vi "Image Browser.vi"() -> ()   [LabVIEW 2014]
doc: "This example shows how to set up an image browser. An image browser is a concise representation of the images in your database represented as thumbnails on a page. You can use the Browser VIs in NI Vision to configure a browser, configure the selection of one or many images, add new images and remove images to and from a browser, replace an image, and get or set the selection status of an image."
uses:
  <vilib>/vision/NI_Vision_Development_Module.lvlib
panel:
  out "Image":T1(plugin-control)
  in  "Stop":bool
  # "Overview: Demonstrates how to use the IMAQ Browser functions to display multiple thumbnail images in a single display. and allow the user to select images from the browser.\nRequirements: Vision Development Software.\nInstructions:\n1. Run the VI.\n2. Click on the images to select or unselect them."
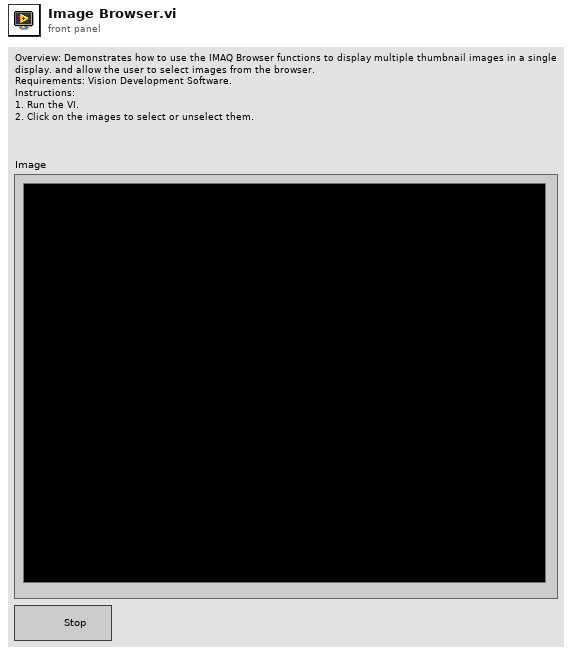
[diagram p1: front panel]
types:
  T1 = typedef "IMAQ Image.ctl" = refnum<image>
  T2 = cluster{"Browser Size":cluster{"X":i32, "Y":i32}, "Images per Line":i32, "Background Color":u32, "Frame Size":i32, "Frame Style":u16}
  T3 = typedef "Image Type" = u32
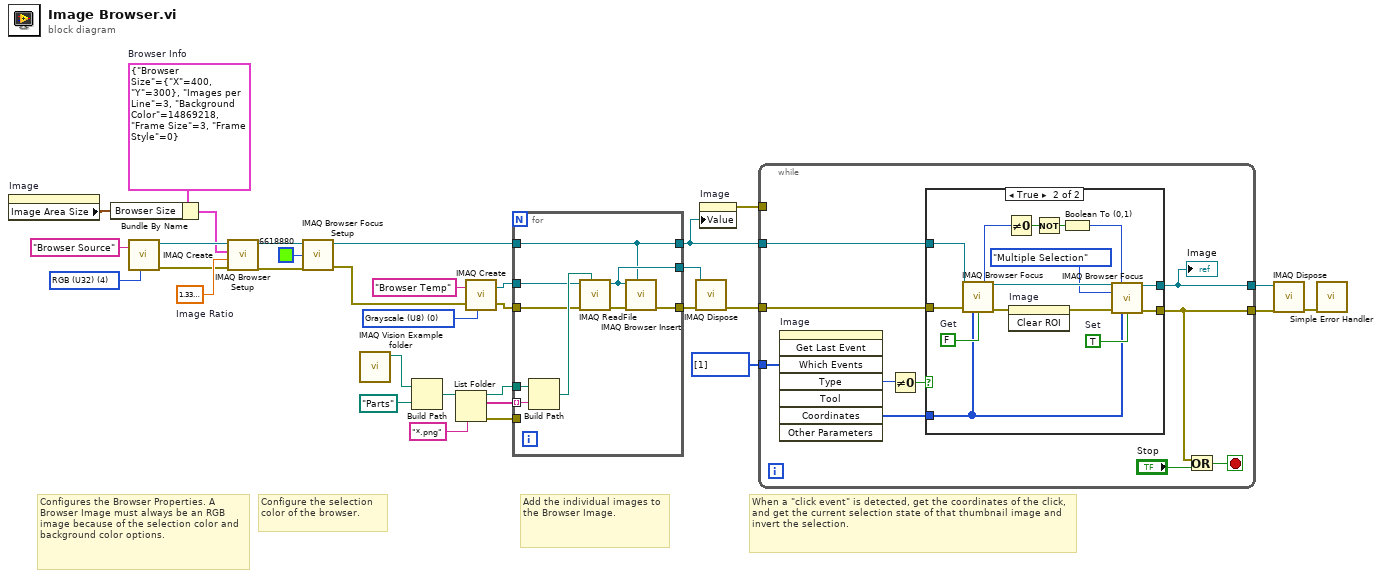
[diagram p0: block diagram]
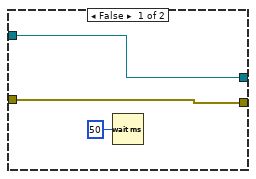
[diagram p2: hidden frame]
diagram:
  w17 = i32[] [1] items=["No Event"=0, "Click Event"=1, "Draw Event"=2, "Size Event"=4, "Scroll Event"=5, "Double Click Event"=8] ("Which Events")
  w33 = sgl 1.33  # Image Ratio
  w5 = T2 {"Browser Size"={"X"=400, "Y"=300}, "Images per Line"=3, "Background Color"=14869218, "Frame Size"=3, "Frame Style"=0}  # Browser Info
  w21 = T3 0 items=["Grayscale (U8)", "Grayscale (I16)", "Grayscale (SGL)", "Complex (CSG)", "RGB (U32)", "HSL (U32)", "RGB (U64)", "Grayscale (U16)"] ("Image Type")
  w23 = T3 4 items=["Grayscale (U8)", "Grayscale (I16)", "Grayscale (SGL)", "Complex (CSG)", "RGB (U32)", "HSL (U32)", "RGB (U64)", "Grayscale (U16)"] ("Image Type")
  # "When a \"click event\" is detected, get the coordinates of the click, and get the current selection state of that thumbnail image and invert the selection."
  # "Add the individual images to the Browser Image."
  # "Configure the selection color of the browser."
  # "Configures the Browser Properties. A Browser Image must always be an RGB image because of the selection color and background color options."
  n1 = property on="Image" class="ImageControl"() -> ("Image Area Size"=w4:cluster{"Width":u32, "Height":u32})  [unwired: 2 in, 2 out]
  n2 = Bundle By Name(cluster=w5, "Browser Size"=w4) -> (w3:T2)
  n3 = call "IMAQ Create"("Image Name"="Browser Source", "Image Type"=w23) -> ("New Image"=w25:T1, "error out"=w24:errorcluster)  [unwired: 3 in]
  n4 = call "IMAQ Browser Setup"("error in (no error)"=w24, "Image Ratio"=w33, "Browser Info"=w3, "Image In"=w25) -> ("error out"=w9:errorcluster, "Image Browser Out"=w10:T1)  [unwired: 2 out]
  n5 = call "IMAQ Browser Focus Setup"("error in (no error)"=w9, "Focus Color"=u32 6618880, "Image Browser In"=w10) -> ("error out"=w7:errorcluster, "Image Browser Out"=w8:T1)  [unwired: 1 in]
  n6 = call "IMAQ Vision Example folder.vi"() -> ("Example Image Path"=w32:path)  [unwired: 11 in]
  n7 = Build Path(base path=w32, name or relative path=path "Parts" ("prompt")) -> (appended path=w28:path)
  n8 = List Folder(path=w28, pattern="*.png") -> (path out=w27:path, filenames=w26:string[], error out=w1:errorcluster)  [unwired: 2 in, 1 out]
  n9 = call "IMAQ Create"("Image Name"="Browser Temp", "Image Type"=w21, "error in (no error)"=w7) -> ("New Image"=w13:T1, "error out"=w30:errorcluster)  [unwired: 2 in]
  n10 = for {
    tunnel: w8 -> [w34]
    tunnel: w27 -> [w42]
    tunnel: w26 -> [w39] mode=indexing
    tunnel: w30 -> [w38]
    tunnel: [w37] -> w29
    tunnel: [w34] -> w18
    tunnel: w13 -> [w36]
    tunnel: [w35] -> w12
    tunnel: w1 -> [_]
    n11 = Build Path(base path=w42, name or relative path=w39) -> (appended path=w41:path)
    n12 = call "IMAQ ReadFile"("File Path"=w41, "error in (no error)"=w38, "Image"=w36) -> ("error out"=w40:errorcluster, "Image Out"=w35:T1)  [unwired: 4 in, 3 out]
    n13 = call "IMAQ Browser Insert"("Image Browser In"=w34, "error in (no error)"=w40, "Image to Add"=w35) -> ("error out"=w37:errorcluster)  [unwired: 4 in, 4 out]
  }
  n14 = call "IMAQ Dispose"("Image"=w12, "error in (no error)"=w29) -> ("error out"=w19:errorcluster)  [unwired: 4 in]
  n15 = property on="Image" class="ImageControl"("Value"=w18) -> (error out=w2:errorcluster)  [unwired: 2 in, 1 out]
  n16 = while {
    tunnel: w18 -> [w52]
    tunnel: w19 -> [w49]
    tunnel: w17 -> [w50]
    tunnel: [w47] -> w16
    tunnel: [w44] -> w15
    tunnel: w2 -> [_]
    stop <- w45 stop-if-true
    n17 = invoke on="Image" class="ImageControl" method="Get Last Event"("Which Events"=w50) -> ("Type"=w43:i32, "Coordinates"=w51:i32[])  [unwired: 7 in, 6 out]
    n18 = Not Equal To 0?(x=w43) -> (x != 0?=w48:bool)
    n19 = case shown="True" w48 {
      tunnel: w52 -> [w54 w70]
      tunnel: w51 -> [_ w61]
      tunnel: w49 -> [w55 w60]
      tunnel: [w55 w59] -> w47
      tunnel: [w54 w58] -> w44
      frame False {
        n20 = Wait (ms)(milliseconds to wait=u32 50) -> ()  [unwired: 1 out]
      }
      frame True {
        w68 = TRUE  # Set
        w69 = FALSE  # Get
        n21 = call "IMAQ Browser Focus"("Image Browser In"=w70, "error in (no error)"=w60, "Pixel Position"=w61, "Get/Set (Set)"=w69) -> ("State Out"=w65:enum16{"Not selected", "Selected"}, "Image Browser Out"=w67:T1, "error out"=w57:errorcluster)  [unwired: 6 in, 3 out]
        n22 = Not Equal To 0?(x=w65) -> (x != 0?=w63:bool)
        n23 = invoke on="Image" class="ImageControl" method="Clear ROI"(error in=w57) -> (error out=w56:errorcluster)  [unwired: 2 in, 2 out]
        n24 = Not(x=w63) -> (.not. x?=w62:bool)
        n25 = Boolean To (0,1)(Boolean=w62) -> (0, 1=w64:i16)
        n26 = call "IMAQ Browser Focus"("Image Browser In"=w67, "State In"=w64, "Selection Mode"=enum16{"Single Selection", "Multiple Selection"}."Multiple Selection", "error in (no error)"=w56, "Pixel Position"=w61, "Get/Set (Set)"=w68) -> ("Image Browser Out"=w58:T1, "error out"=w59:errorcluster)  [unwired: 4 in, 4 out]
      }
    }
    "Image" <- w44
    n27 = Or(x=w47, y="Stop") -> (x .or. y?=w45:bool)
  }
  n28 = call "IMAQ Dispose"("Image"=w15, "error in (no error)"=w16) -> ("error out"=w14:errorcluster)  [unwired: 4 in]
  n29 = call <vilib>:"Simple Error Handler.vi"("error in (no error)"=w14) -> ()  [unwired: 4 in, 5 out]
